vi "SpoolToDisk_WithTimestamp.vi"(0 "Handle":i32, 1 "PreAmp Gain Control":string(combo), 2 "ExposureTime":dbl=0.1, 3 "AOI Height":i64, 4 "AOI Width":i64, 5 "Centre AOI":bool, 6 "trigger mode":string(combo), 7 "NumImages":i32=10, 8 "Shutter":string(combo)="Rolling", 10 "Pixel Readout Rate":string(combo)="280 MHz", 12 "Overlap":bool, 14 "ByteData":u8[](array[numeric])) -> (9 "FrameRate":dbl, 11 "ImageSizeBytes":i64)   [LabVIEW 2019]
uses:
  <userlib>/AndorSDK3/Data/GetPixelData16.vi
panel:
  out "Intensity Graph":u16[][](graph)
  out "String":string
  out "MetaData":i64
  out "TimeStamp":dbl
  in  "Apply Settings":bool
  out "Current Image":i32
  in  "Path":path=path "C:/"
  out "Ready":bool
  in  "Run":bool
  in  "error":errorcluster
  out "Pixel Encoding":string
  out "AOIStride":i64
  in  "PixelData":u16[](array[numeric])
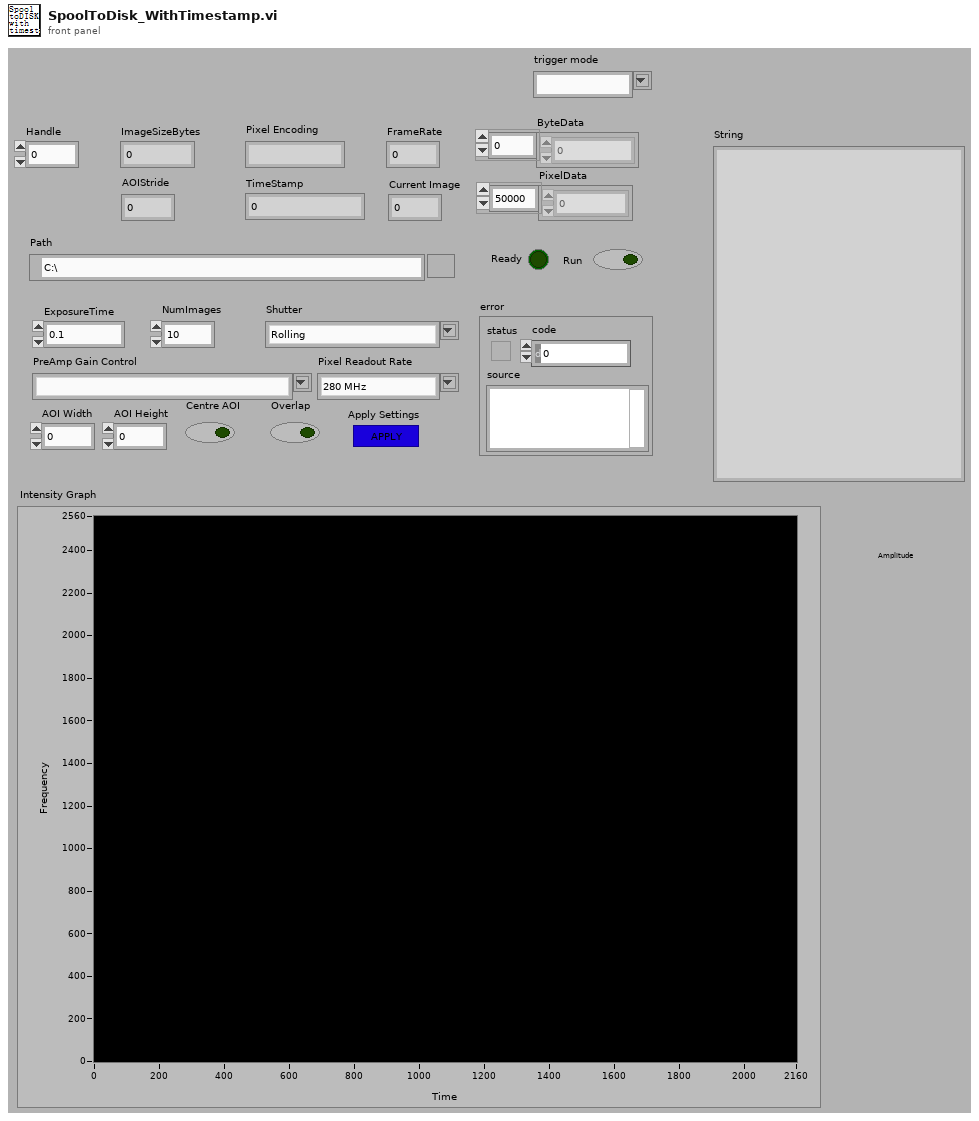
[diagram p1: front panel]
types:
  T1 = enum8{"Enabled", "Disabled", "Disabled and Grayed Out"}
  T2 = enum16{"big-endian, network order", "native, host order", "little-endian"}
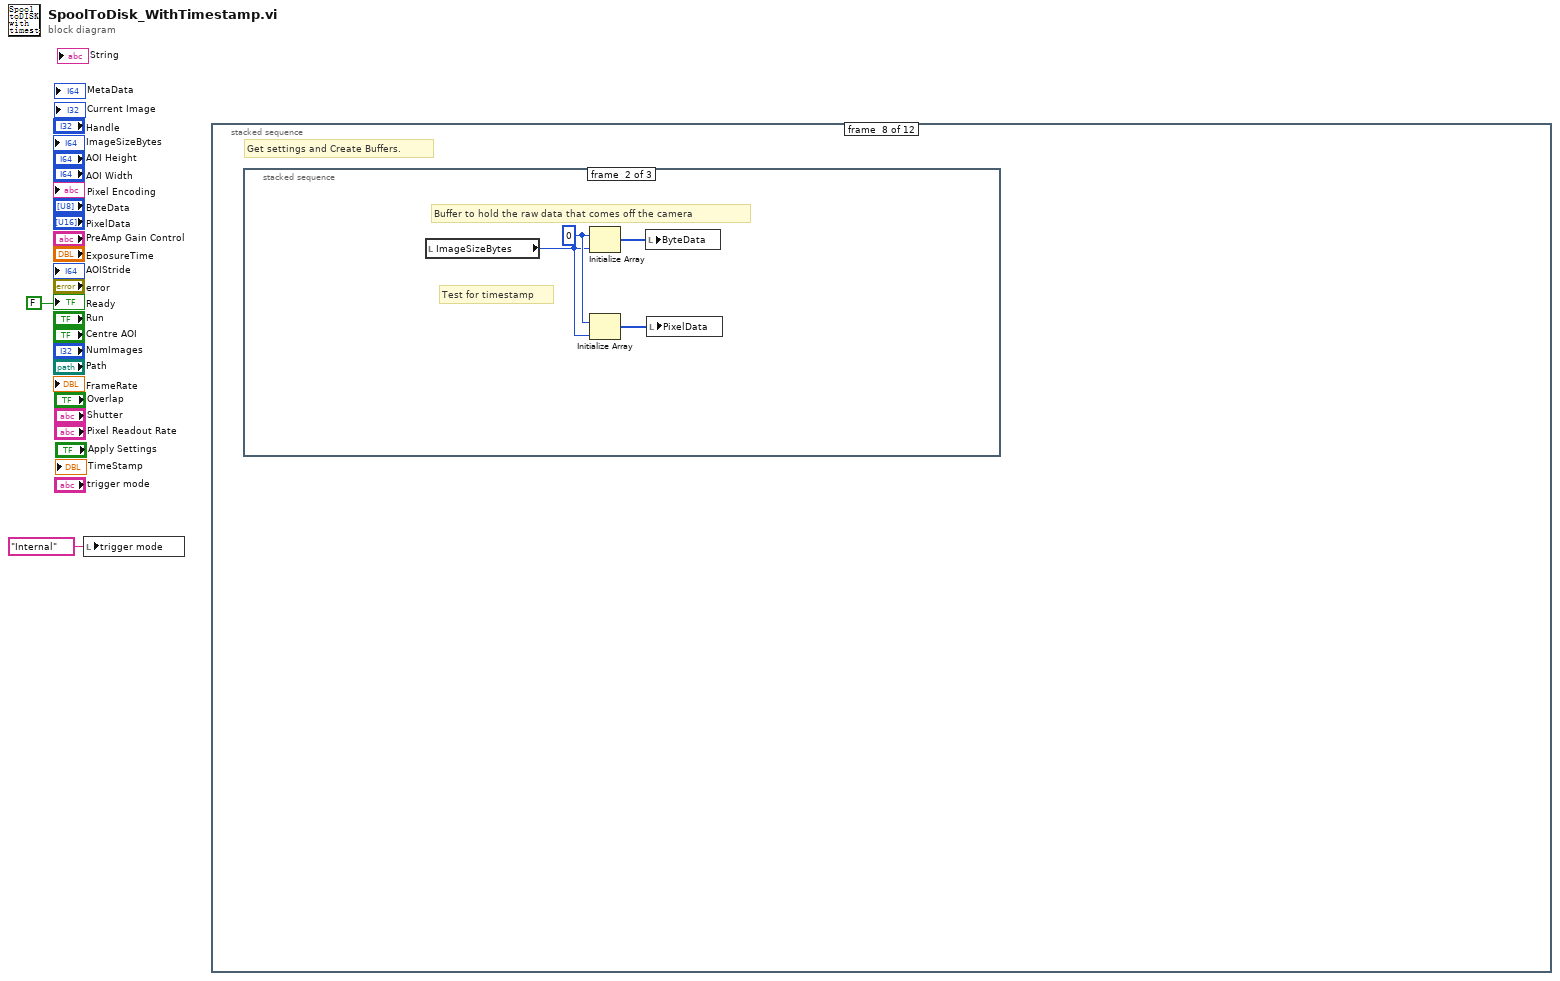
[diagram p0: block diagram]
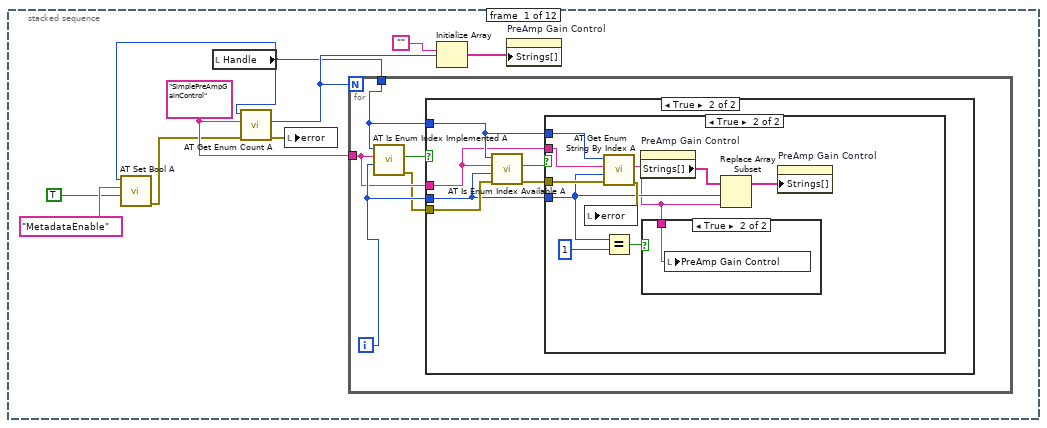
[diagram p2: hidden frame]
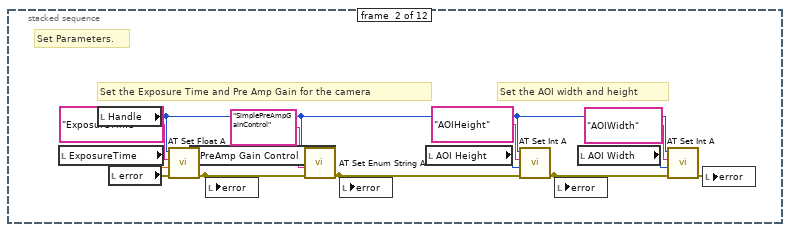
[diagram p6: hidden frame]
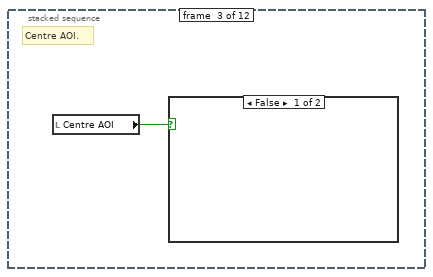
[diagram p7: hidden frame]
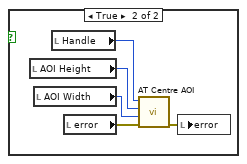
[diagram p8: hidden frame]
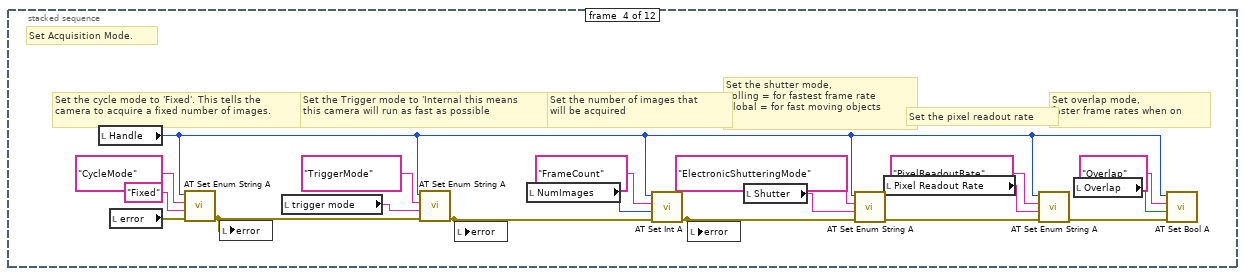
[diagram p9: hidden frame]
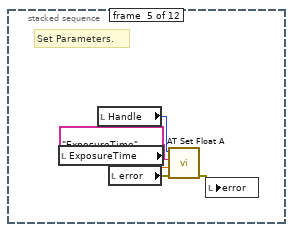
[diagram p10: hidden frame]
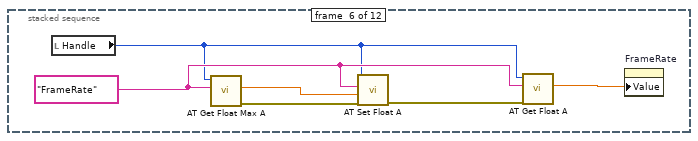
[diagram p11: hidden frame]
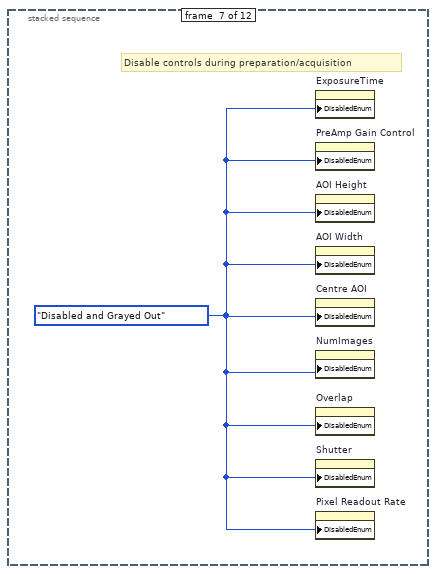
[diagram p12: hidden frame]
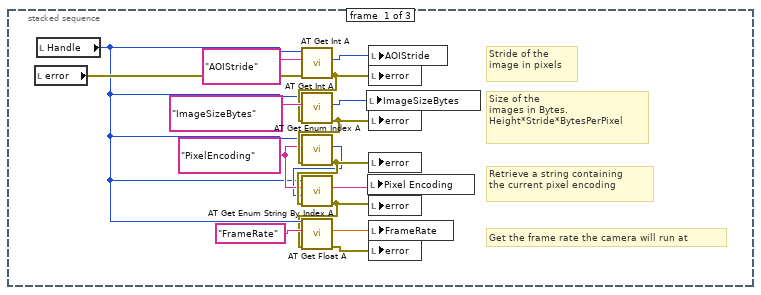
[diagram p13: hidden frame]
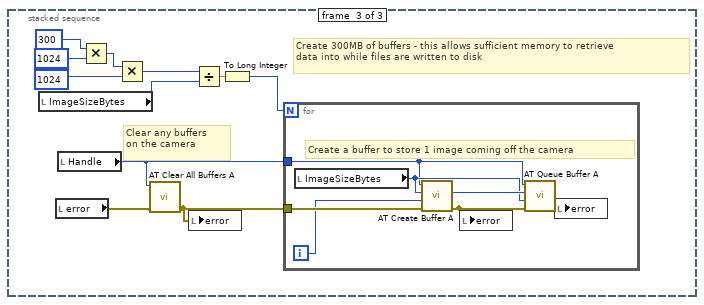
[diagram p14: hidden frame]
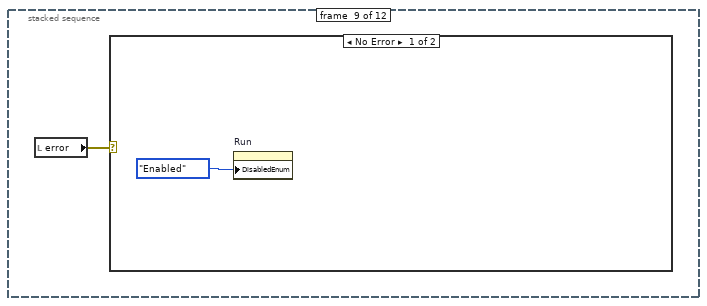
[diagram p15: hidden frame]
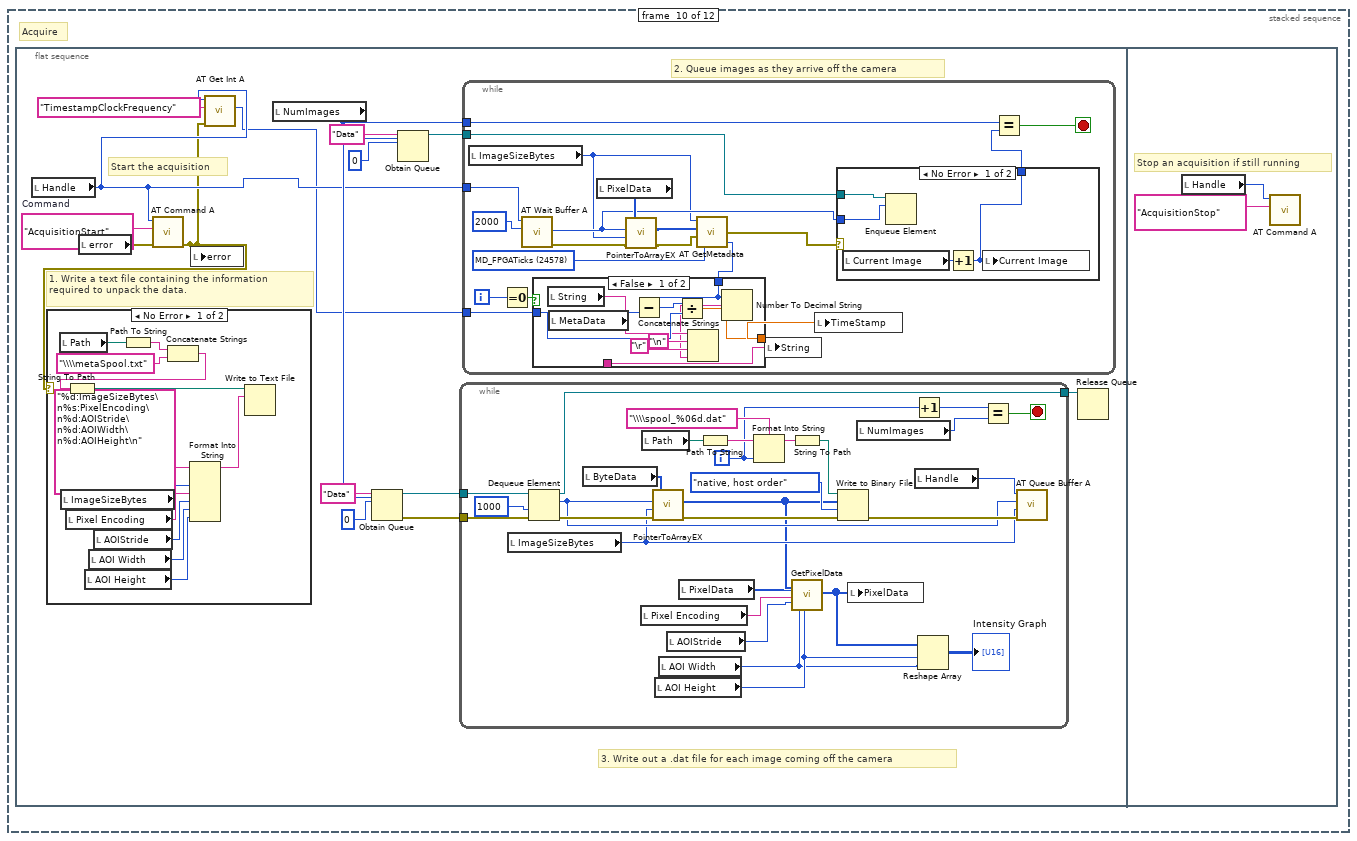
[diagram p17: hidden frame]
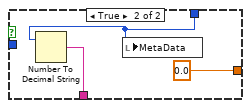
[diagram p18: hidden frame]
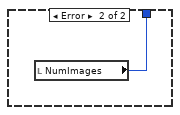
[diagram p19: hidden frame]
diagram:
  n1 = local write "trigger mode"("Internal" ("trigger mode")) -> ()
  n2 = stacked-sequence {
    frame #0 {
      w10 = "SimplePreAmpGainControl" ("SimplePreAmpGainControl")
      n3 = local read "Handle"() -> (w5:i32)
      n4 = call <userlib>:"AT Set Bool A.vi"("Value"=TRUE, "Feature"="MetadataEnable", "Handle"=w5) -> ("error out"=w3:errorcluster)  [unwired: 7 in, 1 out]
      n5 = call <userlib>:"AT Get Enum Count A.vi"("error in (no error)"=w3, "Feature"=w10, "Handle"=w5) -> ("error out"=w11:errorcluster, "Count"=w9:i32)  [unwired: 6 in, 1 out]
      n6 = local write "error"(w11) -> ()
      n7 = for {
        N: w9 -> [_]
        tunnel: w5 -> [w13]
        tunnel: w10 -> [w14]
        i -> [w15]
        n8 = call <userlib>:"AT Is Enum Index Implemented A.vi"("Index"=w15, "Feature"=w14, "Handle"=w13) -> ("error out"=w12:errorcluster, "Implemented"=w16:bool)  [unwired: 6 in, 1 out]
        n9 = case shown="True" w16 {
          tunnel: w15 -> [_ w18]
          tunnel: w14 -> [_ w19]
          tunnel: w13 -> [_ w20]
          tunnel: w12 -> [_ w22]
          frame False {
          }
          frame True {
            n10 = call <userlib>:"AT Is Enum Index Available A.vi"("error in (no error)"=w22, "Index"=w18, "Feature"=w19, "Handle"=w20) -> ("error out"=w17:errorcluster, "Available"=w21:bool)  [unwired: 5 in, 1 out]
            n11 = case shown="True" w21 {
              tunnel: w20 -> [_ w32]
              tunnel: w19 -> [_ w31]
              tunnel: w18 -> [_ w28]
              tunnel: w17 -> [_ w30]
              frame False {
              }
              frame True {
                n12 = call <userlib>:"AT Get Enum String By Index A.vi"("error in (no error)"=w30, "Index"=w28, "Feature"=w31, "Handle"=w32) -> ("error out"=w29:errorcluster, "String"=w25:string)  [unwired: 5 in, 1 out]
                n13 = local write "error"(w29) -> ()
                n14 = Equal?(x=w28, y=1) -> (x = y?=w26:bool)
                n15 = property on="PreAmp Gain Control" class="CmbBox"() -> ("Strings[]"=w24:string[])  [unwired: 2 in, 2 out]
                n16 = case shown="True" w26 {
                  tunnel: w25 -> [_ w33]
                  frame False {
                  }
                  frame True {
                    n17 = local write "PreAmp Gain Control"(w33) -> ()
                  }
                }
                n18 = Replace Array Subset(array=w24, new element=w25, index=w28) -> (w23:string[])
                n19 = property on="PreAmp Gain Control" class="CmbBox"("Strings[]"=w23) -> ()  [unwired: 2 in, 2 out]
              }
            }
          }
        }
      }
      n20 = Initialize Array("", w9) -> (w7:string[])
      n21 = property on="PreAmp Gain Control" class="CmbBox"("Strings[]"=w7) -> ()  [unwired: 2 in, 2 out]
    }
    frame #1 {
      # "Set the AOI width and height"
      # "Set the Exposure Time and Pre Amp Gain for the camera"
      # "Set Parameters."
      n22 = local read "ExposureTime"() -> (w47:dbl)
      n23 = local read "Handle"() -> (w34:i32)
      n24 = local read "error"() -> (w42:errorcluster)
      n25 = call <userlib>:"AT Set Float A.vi"("error in (no error)"=w42, "Value"=w47, "Feature"="ExposureTime" ("ExposureTime"), "Hndl"=w34) -> ("error out"=w45:errorcluster)  [unwired: 6 in, 1 out]
      n26 = local read "PreAmp Gain Control"() -> (w46:string)
      n27 = local write "error"(w45) -> ()
      n28 = call <userlib>:"AT Set Enum String A.vi"("error in (no error)"=w45, "String"=w46, "Feature"="SimplePreAmpGainControl" ("SimplePreAmpGainControl"), "Handle"=w34) -> ("error out"=w41:errorcluster)  [unwired: 6 in, 1 out]
      n29 = local write "error"(w41) -> ()
      n30 = local read "AOI Height"() -> (w38:i64)
      n31 = call <userlib>:"AT Set Int A.vi"("error in (no error)"=w41, "Value"=w38, "Feature"="AOIHeight" ("Integer feature"), "Handle"=w34) -> ("error out"=w39:errorcluster)  [unwired: 6 in, 1 out]
      n32 = local write "error"(w39) -> ()
      n33 = local read "AOI Width"() -> (w37:i64)
      n34 = call <userlib>:"AT Set Int A.vi"("error in (no error)"=w39, "Value"=w37, "Feature"="AOIWidth" ("Integer feature 2"), "Handle"=w34) -> ("error out"=w40:errorcluster)  [unwired: 6 in, 1 out]
      n35 = local write "error"(w40) -> ()
    }
    frame #2 {
      # "Centre AOI."
      n36 = local read "Centre AOI"() -> (w48:bool)
      n37 = case shown="False" w48 {
        frame False {
        }
        frame True {
          n38 = local read "AOI Height"() -> (w50:i64)
          n39 = local read "AOI Width"() -> (w51:i64)
          n40 = local read "Handle"() -> (w49:i32)
          n41 = local read "error"() -> (w52:errorcluster)
          n42 = call <userlib>:"AT Centre AOI.vi"("error in (no error)"=w52, "AOI Width"=w51, "AOI Height"=w50, "Handle"=w49) -> ("error out"=w53:errorcluster)  [unwired: 7 in]
          n43 = local write "error"(w53) -> ()
        }
      }
    }
    frame #3 {
      # "Set overlap mode,\nfaster frame rates when on"
      # "Set the pixel readout rate"
      # "Set the shutter mode,\nRolling = for fastest frame rate\nGlobal = for fast moving objects"
      # "Set the number of images that \nwill be acquired"
      # "Set the Trigger mode to 'Internal this means \nthis camera will run as fast as possible"
      # "Set the cycle mode to 'Fixed'. This tells the \ncamera to acquire a fixed number of images."
      # "Set Acquisition Mode."
      n44 = local read "Handle"() -> (w60:i32)
      n45 = local read "error"() -> (w70:errorcluster)
      n46 = call <userlib>:"AT Set Enum String A.vi"("error in (no error)"=w70, "String"="Fixed", "Feature"="CycleMode" ("Enum feature"), "Handle"=w60) -> ("error out"=w69:errorcluster)  [unwired: 6 in, 1 out]
      n47 = local write "error"(w69) -> ()
      n48 = local read "trigger mode"() -> (w54:string)
      n49 = call <userlib>:"AT Set Enum String A.vi"("error in (no error)"=w69, "String"=w54, "Feature"="TriggerMode" ("Enum feature"), "Handle"=w60) -> ("error out"=w67:errorcluster)  [unwired: 6 in, 1 out]
      n50 = local write "error"(w67) -> ()
      n51 = local read "NumImages"() -> (w65:i32)
      n52 = call <userlib>:"AT Set Int A.vi"("error in (no error)"=w67, "Value"=w65, "Feature"="FrameCount" ("Integer feature 2"), "Handle"=w60) -> ("error out"=w64:errorcluster)  [unwired: 6 in, 1 out]
      n53 = local write "error"(w64) -> ()
      n54 = local read "Shutter"() -> (w57:string)
      n55 = call <userlib>:"AT Set Enum String A.vi"("error in (no error)"=w64, "String"=w57, "Feature"="ElectronicShutteringMode" ("ElectronicShutteringMode"), "Handle"=w60) -> ("error out"=w63:errorcluster)  [unwired: 6 in, 1 out]
      n56 = local read "Pixel Readout Rate"() -> (w56:string)
      n57 = call <userlib>:"AT Set Enum String A.vi"("error in (no error)"=w63, "String"=w56, "Feature"="PixelReadoutRate" ("PixelReadoutRate"), "Handle"=w60) -> ("error out"=w62:errorcluster)  [unwired: 6 in, 1 out]
      n58 = local read "Overlap"() -> (w55:bool)
      n59 = call <userlib>:"AT Set Bool A.vi"("error in (no error)"=w62, "Value"=w55, "Feature"="Overlap" ("Overlap"), "Handle"=w60) -> ()  [unwired: 6 in, 2 out]
    }
    frame #4 {
      # "Set Parameters."
      n60 = local read "ExposureTime"() -> (w77:dbl)
      n61 = local read "Handle"() -> (w73:i32)
      n62 = local read "error"() -> (w74:errorcluster)
      n63 = call <userlib>:"AT Set Float A.vi"("error in (no error)"=w74, "Value"=w77, "Feature"="ExposureTime" ("ExposureTime"), "Hndl"=w73) -> ("error out"=w76:errorcluster)  [unwired: 6 in, 1 out]
      n64 = local write "error"(w76) -> ()
    }
    frame #5 {
      w80 = "FrameRate" ("FrameRate")
      n65 = local read "Handle"() -> (w79:i32)
      n66 = call <userlib>:"AT Get Float Max A.vi"("Feature"=w80, "Handle"=w79) -> ("error out"=w83:errorcluster, "MaxValue"=w82:dbl)  [unwired: 7 in, 1 out]
      n67 = call <userlib>:"AT Set Float A.vi"("error in (no error)"=w83, "Value"=w82, "Feature"=w80, "Hndl"=w79) -> ("error out"=w81:errorcluster)  [unwired: 6 in, 1 out]
      n68 = call <userlib>:"AT Get Float A.vi"("error in (no error)"=w81, "Feature"=w80, "Handle"=w79) -> ("Value"=w78:dbl)  [unwired: 6 in, 2 out]
      n69 = property on="FrameRate" class="DigNum (strict)"("Value"=w78) -> ()  [unwired: 2 in, 2 out]
    }
    frame #6 {
      w84 = T1."Disabled and Grayed Out" ("Disabled")
      # "Disable controls during preparation/acquisition"
      n70 = property on="ExposureTime" class="DigNum (strict)"("DisabledEnum"=w84) -> ()  [unwired: 2 in, 2 out]
      n71 = property on="PreAmp Gain Control" class="CmbBox"("DisabledEnum"=w84) -> ()  [unwired: 2 in, 2 out]
      n72 = property on="AOI Height" class="DigNum (strict)"("DisabledEnum"=w84) -> ()  [unwired: 2 in, 2 out]
      n73 = property on="AOI Width" class="DigNum (strict)"("DisabledEnum"=w84) -> ()  [unwired: 2 in, 2 out]
      n74 = property on="Centre AOI" class="Bool (strict)"("DisabledEnum"=w84) -> ()  [unwired: 2 in, 2 out]
      n75 = property on="NumImages" class="DigNum (strict)"("DisabledEnum"=w84) -> ()  [unwired: 2 in, 2 out]
      n76 = property on="Overlap" class="Bool (strict)"("DisabledEnum"=w84) -> ()  [unwired: 2 in, 2 out]
      n77 = property on="Shutter" class="CmbBox"("DisabledEnum"=w84) -> ()  [unwired: 2 in, 2 out]
      n78 = property on="Pixel Readout Rate" class="CmbBox"("DisabledEnum"=w84) -> ()  [unwired: 2 in, 2 out]
    }
    frame #7 {
      # "Get settings and Create Buffers."
      n79 = stacked-sequence {
        frame #0 {
          w93 = "PixelEncoding" ("Enum feature")
          # "Get the frame rate the camera will run at"
          # "Retrieve a string containing \nthe current pixel encoding"
          # "Stride of the\nimage in pixels"
          # "Size of the\nimages in Bytes.\nHeight*Stride*BytesPerPixel"
          n80 = local read "error"() -> (w90:errorcluster)
          n81 = local read "Handle"() -> (w87:i32)
          n82 = call <userlib>:"AT Get Int A.vi"("error in (no error)"=w90, "Feature"="AOIStride" ("Integer feature"), "Handle"=w87) -> ("error out"=w96:errorcluster, "Value"=w100:i64)  [unwired: 6 in, 1 out]
          n83 = call <userlib>:"AT Get Int A.vi"("error in (no error)"=w96, "Feature"="ImageSizeBytes" ("Integer feature"), "Handle"=w87) -> ("error out"=w95:errorcluster, "Value"=w99:i64)  [unwired: 6 in, 1 out]
          n84 = call <userlib>:"AT Get Enum Index A.vi"("error in (no error)"=w95, "Feature"=w93, "Handle"=w87) -> ("error out"=w94:errorcluster, "Value"=w92:i32)  [unwired: 6 in, 1 out]
          n85 = call <userlib>:"AT Get Enum String By Index A.vi"("error in (no error)"=w94, "Index"=w92, "Feature"=w93, "Handle"=w87) -> ("error out"=w86:errorcluster, "String"=w91:string)  [unwired: 5 in, 1 out]
          n86 = call <userlib>:"AT Get Float A.vi"("error in (no error)"=w86, "Feature"="FrameRate", "Handle"=w87) -> ("error out"=w88:errorcluster, "Value"=w85:dbl)  [unwired: 6 in, 1 out]
          n87 = local write "ImageSizeBytes"(w99) -> ()
          n88 = local write "Pixel Encoding"(w91) -> ()
          n89 = local write "AOIStride"(w100) -> ()
          n90 = local write "error"(w96) -> ()
          n91 = local write "error"(w95) -> ()
          n92 = local write "error"(w94) -> ()
          n93 = local write "error"(w86) -> ()
          n94 = local write "FrameRate"(w85) -> ()
          n95 = local write "error"(w88) -> ()
        }
        frame #1 {
          w102 = u8 0
          # "Test for timestamp"
          # "Buffer to hold the raw data that comes off the camera"
          n96 = local read "ImageSizeBytes"() -> (w101:i64)
          n97 = Initialize Array(w102, w101) -> (w103:u8[])
          n98 = Initialize Array(w102, w101) -> (w104:u8[])
          n99 = local write "ByteData"(w103) -> ()
          n100 = local write "PixelData"(w104) -> ()
        }
        frame #2 {
          # "Create 300MB of buffers - this allows sufficient memory to retrieve \ndata into while files are written to disk"
          # "Clear any buffers \non the camera"
          n101 = local read "ImageSizeBytes"() -> (w108:i64)
          n102 = local read "error"() -> (w115:errorcluster)
          n103 = local read "Handle"() -> (w113:i32)
          n104 = Multiply(x=300, y=1024) -> (x*y=w111:i32)
          n105 = Multiply(x=w111, y=1024) -> (x*y=w107:i32)
          n106 = call <userlib>:"AT Clear All Buffers A.vi"("error in (no error)"=w115, "Handle"=w113) -> ("error out"=w114:errorcluster)  [unwired: 8 in, 1 out]
          n107 = local write "error"(w114) -> ()
          n108 = Divide(x=w107, y=w108) -> (x/y=w106:dbl)
          n109 = To Long Integer(number=w106) -> (32bit integer=w105:i32)
          n110 = for {
            N: w105 -> [_]
            tunnel: w114 -> [w118]
            tunnel: w113 -> [w117]
            i -> [w116]
            # "Create a buffer to store 1 image coming off the camera"
            n111 = local read "ImageSizeBytes"() -> (w120:i64)
            n112 = call <userlib>:"AT Create Buffer A.vi"("error in (no error)"=w118, "Buffer"=w116, "Size"=w120, "Handle"=w117) -> ("error out"=w121:errorcluster, "Buffer out"=w122:u64)  [unwired: 5 in, 1 out]
            n113 = local write "error"(w121) -> ()
            n114 = call <userlib>:"AT Queue Buffer A.vi"("error in (no error)"=w121, "PtrSize"=w120, "Ptr"=w122, "Handle"=w117) -> ("error out"=w119:errorcluster)  [unwired: 6 in, 1 out]
            n115 = local write "error"(w119) -> ()
          }
        }
      }
    }
    frame #8 {
      n116 = local read "error"() -> (w123:errorcluster)
      n117 = case shown="No Error" w123 {
        frame No Error {
          n118 = property on="Run" class="Bool (strict)"("DisabledEnum"=T1."Enabled" ("Disabled")) -> ()  [unwired: 2 in, 2 out]
        }
        frame Error {
        }
      }
    }
    frame #9 {
      # "Acquire"
      n119 = flat-sequence {
        frame #0 {
          w138 = "AcquisitionStart"  # Command
          # "2. Queue images as they arrive off the camera"
          # "3. Write out a .dat file for each image coming off the camera"
          # "1. Write a text file containing the information \nrequired to unpack the data."
          # "Start the acquisition"
          n120 = local read "Handle"() -> (w127:i32)
          n121 = local read "error"() -> (w139:errorcluster)
          n122 = call <userlib>:"AT Command A.vi"("error in (no error)"=w139, "Feature"=w138, "Handle"=w127) -> ("error out"=w125:errorcluster)  [unwired: 7 in, 1 out]
          n123 = case shown="No Error" w125 {
            frame No Error {
              n124 = local read "Path"() -> (w189:path)
              n125 = local read "ImageSizeBytes"() -> (w178:i64)
              n126 = local read "Pixel Encoding"() -> (w179:string)
              n127 = local read "AOI Height"() -> (w182:i64)
              n128 = local read "AOI Width"() -> (w181:i64)
              n129 = local read "AOIStride"() -> (w180:i64)
              n130 = Path To String(path=w189) -> (string=w187:string)
              n131 = Concatenate Strings(w187, "\\\\metaSpool.txt" ("format string")) -> (w186:string)
              n132 = String To Path(string=w186) -> (path=w185:path)
              n133 = Format Into String(format string="%d:ImageSizeBytes\n%s:PixelEncoding\n%d:AOIStride\n%d:AOIWidth\n%d:AOIHeight\n", w178, w179, w180, w181, w182) -> (resulting string=w183:string)  [unwired: 2 in, 1 out]
              n134 = Write to Text File(file (use dialog)=w185, text=w183) -> ()  [unwired: 2 in, 3 out]
            }
            frame Error {
            }
          }
          n135 = local write "error"(w125) -> ()
          n136 = call <userlib>:"AT Get Int A.vi"("error in (no error)"=w125, "Feature"="TimestampClockFrequency", "Handle"=w127) -> ("Value"=w126:i64)  [unwired: 6 in, 2 out]
          n137 = local read "NumImages"() -> (w129:i32)
          n138 = Obtain Queue(max queue size (-1, unlimited)=w129, name (unnamed)="Data", element data type=u64 0) -> (queue out=w133:refnum<queue>, error out=w134:errorcluster)  [unwired: 2 in, 1 out]
          n139 = Obtain Queue(max queue size (-1, unlimited)=w129, name (unnamed)="Data", element data type=u64 0) -> (queue out=w136:refnum<queue>)  [unwired: 2 in, 2 out]
          n140 = while {
            tunnel: w134 -> [w218]
            tunnel: w133 -> [w217]
            tunnel: [w210] -> w130
            i -> [w205]
            stop <- w209 stop-if-true
            n141 = local read "ImageSizeBytes"() -> (w198:i64)
            n142 = Dequeue Element(queue=w217, timeout in ms (-1)=1000, error in (no error)=w218) -> (queue out=w210:refnum<queue>, element=w199:u64, error out=w201:errorcluster)  [unwired: 1 out]
            n143 = local read "ByteData"() -> (w202:u8[])
            n144 = local read "Pixel Encoding"() -> (w195:string)
            n145 = local read "Path"() -> (w215:path)
            n146 = call <userlib>:"PointerToArrayEX.vi"("Array in"=w202, "Pointer In"=w199, "Pointer Size"=w198, "error in (no error)"=w201) -> ("Array out"=w197:u8[], "error out"=w200:errorcluster)  [unwired: 4 in]
            n147 = local read "AOI Height"() -> (w192:i64)
            n148 = local read "AOI Width"() -> (w191:i64)
            n149 = local read "AOIStride"() -> (w194:i64)
            n150 = local read "PixelData"() -> (w196:u16[])
            n151 = Path To String(path=w215) -> (string=w212:string)
            n152 = Format Into String(format string="\\\\spool_%06d.dat", initial string=w212, w205) -> (resulting string=w213:string)  [unwired: 1 in, 1 out]
            n153 = String To Path(string=w213) -> (path=w208:path)
            n154 = call-poly <userlib>:"GetPixelData.vi"("Input buffer"=w197, "Output buffer in"=w196, "Pixel Encoding"=w195, "Stride"=w194, "Width"=w191, "Height"=w192) -> ("Output buffer out"=w193:u16[])  [unwired: 11 in, 2 out]
            n155 = Write to Binary File(file (use dialog)=w208, data=w197, error in=w200, 9:T2."native, host order" ("byte order (0:big-endian, network order)")) -> (error out=w206:errorcluster)  [unwired: 2 in, 2 out]
            n156 = local write "PixelData"(w193) -> ()
            n157 = local read "NumImages"() -> (w203:i32)
            n158 = Increment(x=w205) -> (x+1=w204:i32)
            n159 = local read "Handle"() -> (w211:i32)
            n160 = Reshape Array(w193, w192, w191) -> (→"Intensity Graph":u16[][])
            n161 = Equal?(x=w204, y=w203) -> (x = y?=w209:bool)
            n162 = call <userlib>:"AT Queue Buffer A.vi"("error in (no error)"=w206, "PtrSize"=w198, "Ptr"=w199, "Handle"=w211) -> ()  [unwired: 6 in, 2 out]
          }
          n163 = while {
            tunnel: w127 -> [w153]
            tunnel: w136 -> [w158]
            tunnel: w129 -> [w157]
            tunnel: w126 -> [w148]
            i -> [w152]
            stop <- w156 stop-if-true
            w147 = u16 24578 items=["MD_FrameData"=24577, "MD_FPGATicks"=24578, "MD_FrameInfo"=24579] ("Metadata Chunk ID")
            n164 = local read "ImageSizeBytes"() -> (w140:i64)
            n165 = Equal To 0?(x=w152) -> (x = 0?=w151:bool)
            n166 = call <userlib>:"AT Wait Buffer A.vi"("Timeout"=u32 2000, "Handle"=w153) -> ("error out"=w144:errorcluster, "Output buffer"=w141:u64)  [unwired: 6 in, 2 out]
            n167 = local read "PixelData"() -> (w145:u16[])
            n168 = call <userlib>:"PointerToArrayEX.vi"("Array in"=w145, "Pointer In"=w141, "Pointer Size"=w140, "error in (no error)"=w144) -> ("Array out"=w142:u8[], "error out"=w143:errorcluster)  [unwired: 4 in]
            n169 = call <userlib>:"AT GetMetadata.vi"("Metadata Chunk ID"=w147, "error in (no error)"=w143, "Input buffer"=w142, "BufferSize"=w140) -> ("MetaData"=w150:i64, "error out"=w154:errorcluster)  [unwired: 1 out]
            n170 = case shown="False" w151 {
              tunnel: w150 -> [w165 w171]
              tunnel: [w166 0.0 ("element data type")] -> w149
              tunnel: w148 -> [w167 _]
              tunnel: [w160 w170] -> w146
              frame False {
                n171 = local read "String"() -> (w164:string)
                n172 = local read "MetaData"() -> (w169:i64)
                n173 = Subtract(x=w165, y=w169) -> (x-y=w168:i64)
                n174 = Divide(x=w168, y=w167) -> (x/y=w166:dbl)
                n175 = Number To Decimal String(number=w165) -> (decimal integer string=w161:string)  [unwired: 1 in]
                n176 = Concatenate Strings(w164, "\n", "\r", w161) -> (w160:string)
              }
              frame True {
                n177 = Number To Decimal String(number=w171) -> (decimal integer string=w170:string)  [unwired: 1 in]
                n178 = local write "MetaData"(w171) -> ()
              }
            }
            n179 = local write "String"(w146) -> ()
            n180 = local write "TimeStamp"(w149) -> ()
            n181 = case shown="No Error" w154 {
              tunnel: w158 -> [w176 _]
              tunnel: [w174 w177] -> w155
              tunnel: w141 -> [w173 _]
              frame No Error {
                n182 = local read "Current Image"() -> (w175:i32)
                n183 = Enqueue Element(queue=w176, element=w173) -> ()  [unwired: 2 in, 3 out]
                n184 = Increment(x=w175) -> (x+1=w174:i32)
                n185 = local write "Current Image"(w174) -> ()
              }
              frame Error {
                n186 = local read "NumImages"() -> (w177:i32)
              }
            }
            n187 = Equal?(x=w157, y=w155) -> (x = y?=w156:bool)
          }
          n188 = Release Queue(queue=w130) -> ()  [unwired: 2 in, 3 out]
        }
        frame #1 {
          # "Stop an acquisition if still running"
          n189 = local read "Handle"() -> (w220:i32)
          n190 = call <userlib>:"AT Command A.vi"("Feature"="AcquisitionStop" ("Command"), "Handle"=w220) -> ()  [unwired: 8 in, 2 out]
        }
      }
    }
    frame #10 {
      w224 = T1."Enabled" ("Disabled")
      # "Clear any buffers \non the camera"
      # "re-enable controls"
      n191 = property on="AOI Height" class="DigNum (strict)"("DisabledEnum"=w224) -> ()  [unwired: 2 in, 2 out]
      n192 = property on="AOI Width" class="DigNum (strict)"("DisabledEnum"=w224) -> ()  [unwired: 2 in, 2 out]
      n193 = property on="PreAmp Gain Control" class="CmbBox"("DisabledEnum"=w224) -> ()  [unwired: 2 in, 2 out]
      n194 = property on="ExposureTime" class="DigNum (strict)"("DisabledEnum"=w224) -> ()  [unwired: 2 in, 2 out]
      n195 = property on="Centre AOI" class="Bool (strict)"("DisabledEnum"=w224) -> ()  [unwired: 2 in, 2 out]
      n196 = property on="NumImages" class="DigNum (strict)"("DisabledEnum"=w224) -> ()  [unwired: 2 in, 2 out]
      n197 = property on="Overlap" class="Bool (strict)"("DisabledEnum"=w224) -> ()  [unwired: 2 in, 2 out]
      n198 = property on="Pixel Readout Rate" class="CmbBox"("DisabledEnum"=w224) -> ()  [unwired: 2 in, 2 out]
      n199 = property on="Shutter" class="CmbBox"("DisabledEnum"=w224) -> ()  [unwired: 2 in, 2 out]
      n200 = local read "error"() -> (w223:errorcluster)
      n201 = local read "Handle"() -> (w221:i32)
      n202 = call <userlib>:"AT Clear All Buffers A.vi"("error in (no error)"=w223, "Handle"=w221) -> ("error out"=w222:errorcluster)  [unwired: 8 in, 1 out]
      n203 = local write "error"(w222) -> ()
    }
    frame #11 {
      # "ShutDown."
      n204 = local write "Ready"(FALSE ("Ready")) -> ()
      n205 = local write "Apply Settings"(FALSE ("Ready")) -> ()
    }
  }
  "Ready" <- FALSE ("Ready")
